vi "ConfigureSimulatedImage.vi"(8 "error in (no error)":errorcluster, 11 "Camera SN":string) -> (0 "error out":errorcluster, 2 "image":T1(plugin-control))   [LabVIEW 2017, in "IrAcquisition.lvlib"]
uses:
  <vilib>/addons/InsightCM/Devices/Shared/Ir/IrAcquisition/IrAcquisition.lvlib
  <vilib>/vision/Image Controls.llb/IMAQ Image.ctl
  <vilib>/addons/InsightCM/Devices/Shared/Ir/IrAcquisition/subVIs/SimConfigGlobal.vi
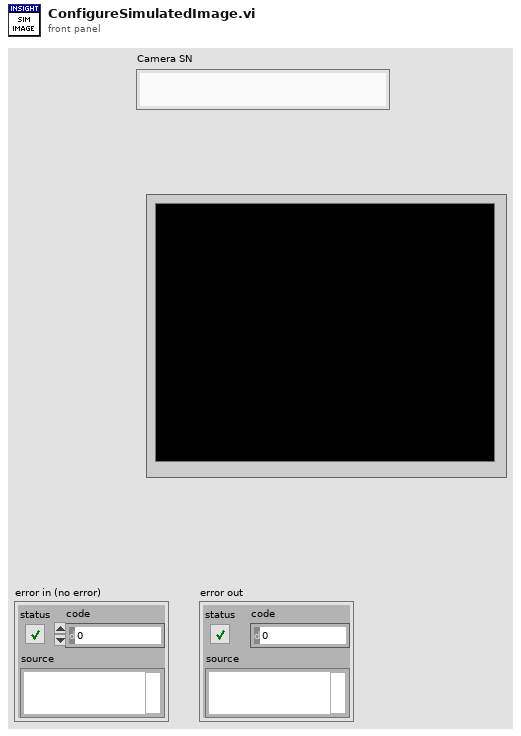
[diagram p1: front panel]
types:
  T1 = typedef "IMAQ Image.ctl" = refnum<image>
  T2 = typedef "Image Type" = u32
  T3 = typedef "simScaleConfig.ctl" = cluster{"Max":cluster{"Enable":bool, "New Max Temp":sgl, "KeepMin":bool}, "Noise":cluster{"Randomize":bool, "Max delta":sgl}, "Hotspot":cluster{"hotspot":bool, "Rectangle":cluster{"left":i16, "top":i16, "right":i16, "bottom":i16}, "Temperature":sgl}}
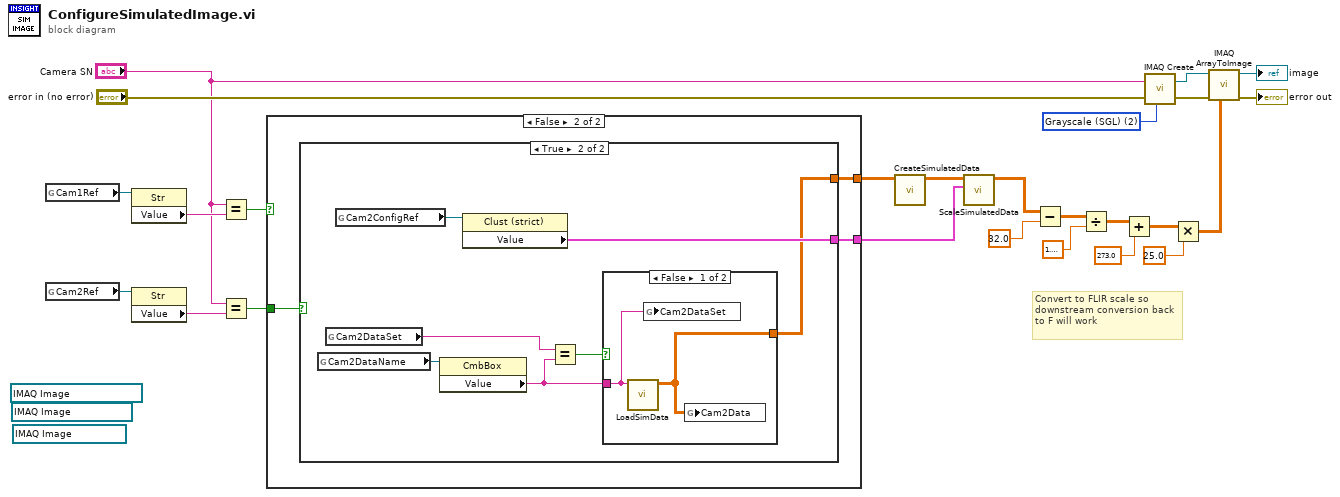
[diagram p0: block diagram]
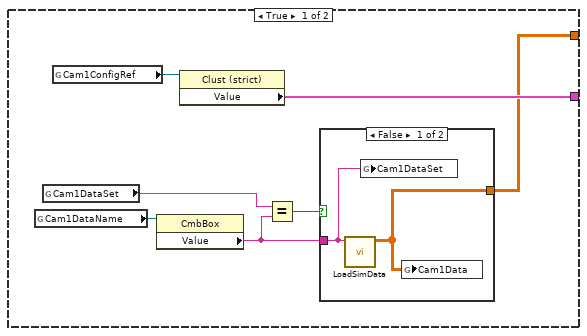
[diagram p2: hidden frame]
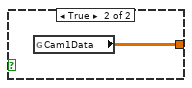
[diagram p3: hidden frame]
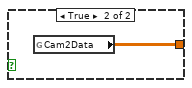
[diagram p5: hidden frame]
diagram:
  w22 = T2 2 items=["Grayscale (U8)", "Grayscale (I16)", "Grayscale (SGL)", "Complex (CSG)", "RGB (U32)", "HSL (U32)", "RGB (U64)", "Grayscale (U16)"] ("Image Type")
  (unwired) T1 refnum ("Original")
  (unwired) T1 refnum ("Original")
  (unwired) T1 refnum ("Original")
  # "Convert to FLIR scale so downstream conversion back to F will work"
  n1 = global read "SimConfigGlobal.vi" "Cam1Ref"() -> (w8:refnum<vi>)
  n2 = global read "SimConfigGlobal.vi" "Cam2Ref"() -> (w3:refnum<vi>)
  n3 = property class="Str"(reference=w8) -> ("Value"=w7:string)  [unwired: 1 in, 2 out]
  n4 = property class="Str"(reference=w3) -> ("Value"=w4:string)  [unwired: 1 in, 2 out]
  n5 = Equal?(x="Camera SN", y=w7) -> (x = y?=w25:bool)
  n6 = Equal?(x="Camera SN", y=w4) -> (x = y?=w1:bool)
  n7 = case shown="False" w25 {
    tunnel: [w31 w38] -> w24
    tunnel: [w27 w37] -> w5
    tunnel: w1 -> [_ w36]
    frame True {
      n8 = global read "SimConfigGlobal.vi" "Cam1DataName"() -> (w30:refnum<vi>)
      n9 = global read "SimConfigGlobal.vi" "Cam1DataSet"() -> (w29:string)
      n10 = global read "SimConfigGlobal.vi" "Cam1ConfigRef"() -> (w32:refnum<vi>)
      n11 = property class="CmbBox"(reference=w30) -> ("Value"=w26:string)  [unwired: 1 in, 2 out]
      n12 = property class="Clust (strict)"(reference=w32) -> ("Value"=w31:T3)  [unwired: 1 in, 2 out]
      n13 = Equal?(x=w29, y=w26) -> (x = y?=w28:bool)
      n14 = case shown="False" w28 {
        tunnel: [w34 w35] -> w27
        tunnel: w26 -> [w33 _]
        frame False {
          n15 = call <vilib>:"LoadSimData.vi"("filename"=w33) -> ("data"=w34:sgl[][])  [unwired: 10 in]
          n16 = global write "SimConfigGlobal.vi" "Cam1DataSet"(w33) -> ()
          n17 = global write "SimConfigGlobal.vi" "Cam1Data"(w34) -> ()
        }
        frame True {
          n18 = global read "SimConfigGlobal.vi" "Cam1Data"() -> (w35:sgl[][])
        }
      }
    }
    frame False {
      n19 = case shown="True" w36 {
        tunnel: [_ w44] -> w38
        tunnel: [_ w40] -> w37
        frame False {
        }
        frame True {
          n20 = global read "SimConfigGlobal.vi" "Cam2DataName"() -> (w43:refnum<vi>)
          n21 = global read "SimConfigGlobal.vi" "Cam2DataSet"() -> (w42:string)
          n22 = global read "SimConfigGlobal.vi" "Cam2ConfigRef"() -> (w45:refnum<vi>)
          n23 = property class="CmbBox"(reference=w43) -> ("Value"=w39:string)  [unwired: 1 in, 2 out]
          n24 = property class="Clust (strict)"(reference=w45) -> ("Value"=w44:T3)  [unwired: 1 in, 2 out]
          n25 = Equal?(x=w42, y=w39) -> (x = y?=w41:bool)
          n26 = case shown="False" w41 {
            tunnel: [w47 w48] -> w40
            tunnel: w39 -> [w46 _]
            frame False {
              n27 = call <vilib>:"LoadSimData.vi"("filename"=w46) -> ("data"=w47:sgl[][])  [unwired: 10 in]
              n28 = global write "SimConfigGlobal.vi" "Cam2DataSet"(w46) -> ()
              n29 = global write "SimConfigGlobal.vi" "Cam2Data"(w47) -> ()
            }
            frame True {
              n30 = global read "SimConfigGlobal.vi" "Cam2Data"() -> (w48:sgl[][])
            }
          }
        }
      }
    }
  }
  n31 = call <vilib>:"CreateSimulatedData.vi"("data in"=w5) -> ("data out"=w6:sgl[][])  [unwired: 10 in]
  n32 = call <vilib>:"ScaleSimulatedData.vi"("Config"=w24, "data in"=w6) -> ("data out"=w10:sgl[][])  [unwired: 9 in]
  n33 = Subtract(x=w10, y=sgl 32.0) -> (x-y=w16:sgl[][])
  n34 = Divide(x=w16, y=sgl 1.8) -> (x/y=w14:sgl[][])
  n35 = Add(x=w14, y=sgl 273.0) -> (x+y=w12:sgl[][])
  n36 = call "IMAQ Create"("Image Name"="Camera SN", "Image Type"=w22, "error in (no error)"="error in (no error)") -> ("New Image"=w23:T1, "error out"=w20:errorcluster)  [unwired: 2 in]
  n37 = Multiply(x=w12, y=sgl 25.0) -> (x*y=w9:sgl[][])
  n38 = call "IMAQ ArrayToImage"("Image Pixels (Float)"=w9, "error in (no error)"=w20, "Image"=w23) -> ("error out"=→"error out":errorcluster, "Image Out"=→"image":T1)  [unwired: 7 in]
